vi "Set_output_channel_group.vi"(8 "error in (no error)":errorcluster, 9 "Group_output":T1, 10 "Channel_output":dbl[](array[numeric]), 11 "_Driver_interaction in":refnum<class "_Driver_interaction.lvclass">) -> (0 "error out":errorcluster, 3 "_Driver_interaction out":refnum<class "_Driver_interaction.lvclass">)   [LabVIEW 2014, in "Driver_interaction.lvlib" / "_Driver_interaction.lvclass"]
uses:
  _Driver_interaction.lvclass
  Toolbox/Controls/Group_output.ctl
  Toolbox/Controls/Group_selector.ctl
  Toolbox/Toolbox.lvclass
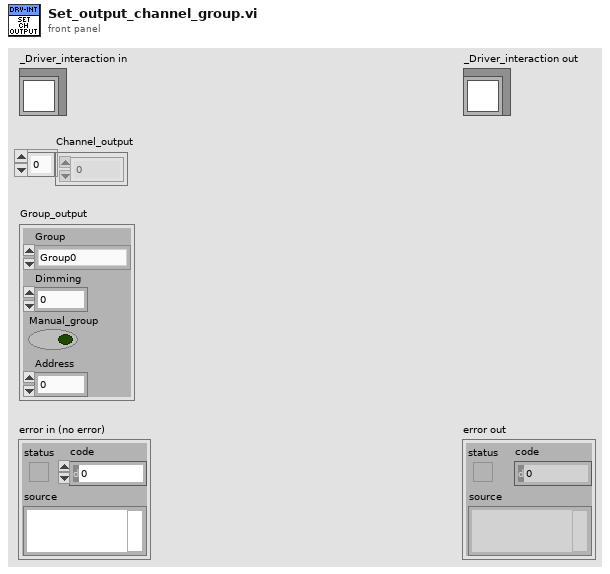
[diagram p1: front panel]
types:
  T1 = typedef "Driver_interaction.lvlib/Toolbox.lvclass/Group_output.ctl" = cluster{"Group":T2, "Dimming":i32, "Manual_group":bool, "Address":i32}
  T2 = typedef "Driver_interaction.lvlib/Toolbox.lvclass/Group_selector.ctl" = enum16{"Group0", "Group1", "Group2", "Group3", "Group4", "Group5", "Group6", "Group7", "Group8", "Group9", "Group10", "Group11", "Group12", "Group13", "Group14", "Group15", "All Groups"}
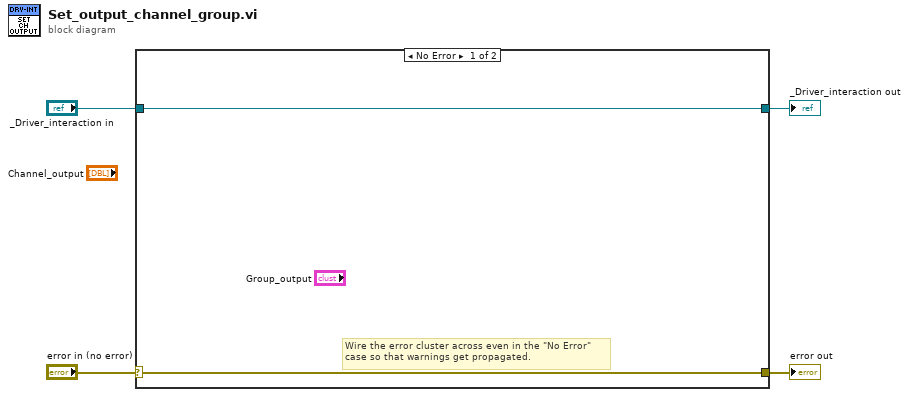
[diagram p0: block diagram]
diagram:
  n1 = case shown="No Error" "error in (no error)" {
    selector: "error in (no error)" -> [w5 w8]
    tunnel: [w5 w8] -> w3
    tunnel: [w6 w7] -> w1
    tunnel: "_Driver_interaction in" -> [w6 w7]
    frame No Error {
      # "Wire the error cluster across even in the \"No Error\"\ncase so that warnings get propagated."
    }
    frame Error {
    }
  }
  "error out" <- w3
  "_Driver_interaction out" <- w1
